vi "ALTS-2015 Set Test Type 1.vi"(8 "error in":errorcluster) -> (0 "error out":errorcluster)   [LabVIEW 2013]
uses:
  Controls/ALTS-2015 LV2GBL Station Info Options.ctl
  Controls/ALTS-2015 LV2GBL Options.ctl
  Controls/ALTS-2015 Station Cluster.ctl
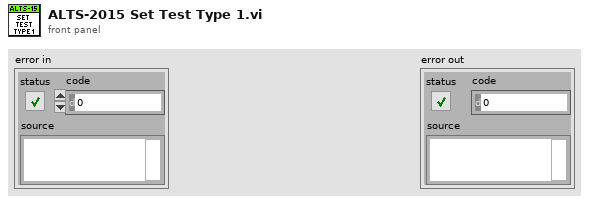
[diagram p1: front panel]
types:
  T1 = typedef "ALTS-2015 Station Cluster.ctl" = enum16{"Station 1", "Station 2", "Station 3", "Station 4"}
  T2 = typedef "ALTS-2015 LV2GBL Options.ctl" = enum16{"Read all", "Write all"}
  T3 = typedef "ALTS-2015 LV2GBL Station Info Options.ctl" = enum16{"Init", "Read", "Read All", "Write Sensor ID", "Write  Work Order", "Write Serial Number", "Write Test Data", "Write Station Status", "Write Station Occupancy", "Write Station Test Type", "Write Rerun", "Write Load Decision", "Write Robot Action", "Clear All", "Clear Test Result"}
  T4 = typedef "ALTS-2015 Station Details.ctl" = cluster{"Station Number":string, "Work Order Number":string, "Sensor Name":string, "Pressure (PSI)":string, "Flow (SCCM)":string, "Test Time ":string, "Test Result":string, "Serial Number":string, "Station Status":T5, "SW assigned UUT":bool, "Rerun Count":i32, "Test Type":i32, "Load Decision":i32, "Robot Action":T6}
  T5 = typedef "ALTS-2015 Status Ring Indicator.ctl" = u16
  T6 = typedef "ALTS-2015 Robot Actions.ctl" = enum16{"Loading...", "Unloading...", "Reruning...", "No Action"}
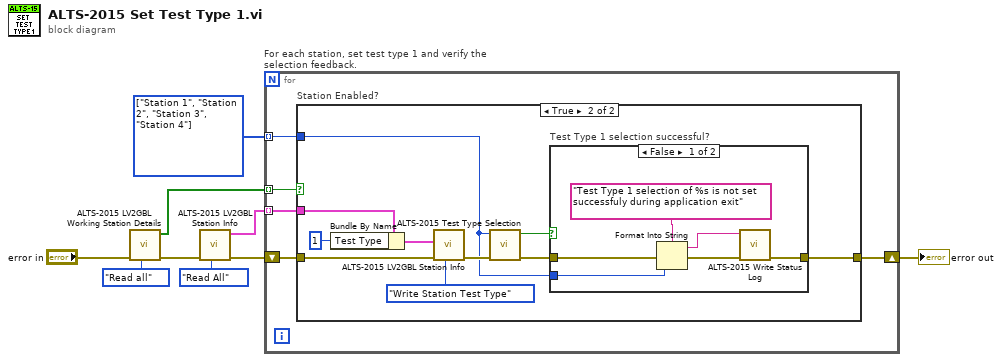
[diagram p0: block diagram]
diagram:
  w7 = T1[] [enum."Station 1", enum."Station 2", enum."Station 3", enum."Station 4"] items=["Station 1", "Station 2", "Station 3", "Station 4"]
  n1 = call "ALTS-2015 LV2GBL Working Station Details.vi"("Options"=ALTS-2015_LV2GBL_Options."Read all", "error in"="error in") -> ("error out"=w4:errorcluster, "Station  Enable Array"=w6:bool[])  [unwired: 8 in]
  n2 = call "ALTS-2015 LV2GBL Station Info.vi"("Options"=ALTS-2015_LV2GBL_Station_Info_Options."Read All", "error in"=w4) -> ("error out"=w3:errorcluster, "Station Info Array"=w2:T4[])  [unwired: 7 in, 1 out]
  n3 = for "For each station, set test type 1 and verify the selection feedback." {
    tunnel: w2 -> [w14] mode=indexing
    shift-right: [w12] -> w9
    shift-left: w3 -> [w13]
    tunnel: w6 -> [w10] mode=indexing
    tunnel: w7 -> [w11] mode=indexing
    n4 = case "Station Enabled?" shown="True" w10 {
      tunnel: w14 -> [_ w24]
      tunnel: w13 -> [w15 w21]
      tunnel: [w15 w18] -> w12
      tunnel: w11 -> [_ w16]
      frame False {
      }
      frame True {
        n5 = Bundle By Name(cluster=w24, "Test Type"=1) -> (w22:T4)
        n6 = call "ALTS-2015 LV2GBL Station Info.vi"("Options"=ALTS-2015_LV2GBL_Station_Info_Options."Write Station Test Type", "error in"=w21, "Station"=w22) -> ("error out"=w20:errorcluster)  [unwired: 6 in, 2 out]
        n7 = call "ALTS-2015 Test Type Selection.vi"("error in (no error)"=w20, "Station Cluster"=w16) -> ("error out"=w19:errorcluster, "Test Type Selection Successful"=w17:bool)  [unwired: 8 in]
        n8 = case "Test Type 1 selection successful?" shown="False" w17 {
          tunnel: w19 -> [w29 w32]
          tunnel: [w28 w32] -> w18
          tunnel: w16 -> [w26 _]
          frame False {
            n9 = Format Into String(format string="Test Type 1 selection of %s is not set successfuly during application exit" ("Status Input"), error in=w29, w26) -> (resulting string=w30:string, error out=w31:errorcluster)  [unwired: 1 in]
            n10 = call "ALTS-2015 Write Status Log.vi"("error in (no error)"=w31, "Status Input"=w30) -> ("error out"=w28:errorcluster)  [unwired: 9 in]
          }
          frame True {
          }
        }
      }
    }
  }
  "error out" <- w9
